vi "Translator.File.GetDefaultStrings (Single).vi"(5 "refnum in":T1, 7 "group":string, 8 "error in":errorcluster, 9 "label":string, 10 "default value":string) -> (0 "error out":errorcluster, 2 "value out":string)   [LabVIEW 2019, in "Tools.lvlib"]
uses:
  Tools.lvlib
  <vilib>/Utility/config.llb/Config Data RefNum.ctl
  <vilib>/Utility/config.llb/Read Key (String).vi
  <vilib>/Utility/config.llb/NI_LVConfig.lvlib
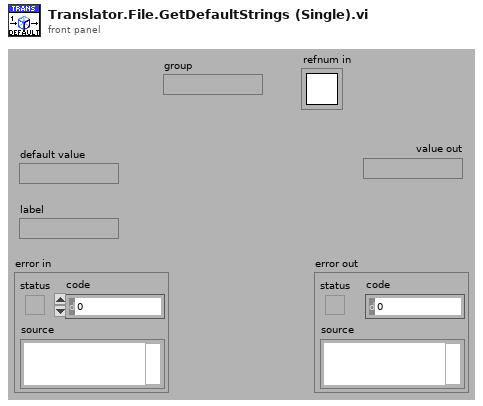
[diagram p1: front panel]
types:
  T1 = typedef "NI_LVConfig.lvlib/Config Data RefNum.ctl" = refnum<k1>
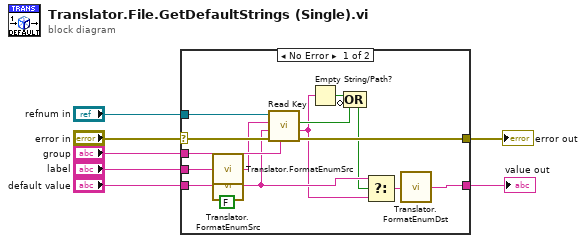
[diagram p0: block diagram]
diagram:
  n1 = case shown="No Error" "error in" {
    selector: "error in" -> [w18 w24]
    tunnel: "refnum in" -> [w17 _]
    tunnel: [w22 w24] -> w7
    tunnel: [w21 w23] -> w4
    tunnel: "group" -> [w20 _]
    tunnel: "label" -> [w16 _]
    tunnel: "default value" -> [w19 w23]
    frame No Error {
      n2 = call "Translator.FormatEnumSrc.vi"("text in"=w16) -> ("text out"=w9:string)  [unwired: 1 in]
      n3 = call "Translator.FormatEnumSrc.vi"("text in"=w19, "quotas?(T)"=FALSE) -> ("text out"=w15:string)
      n4 = call-poly <vilib>:"Read Key.vi"("section"=w20, "error in (no error)"=w18, "default value"=w15, "key"=w9, "refnum"=w17) -> ("error out"=w22:errorcluster, "value"=w11:string, "found?"=w12:bool)  [unwired: 3 in, 1 out]
      n5 = Empty String/Path?(string/path=w11) -> (empty?=w14:bool)
      n6 = Compound Arithmetic op=OR(w14, invert w12) -> (w13:bool)
      n7 = Select(t=w15, s=w13, f=w11) -> (s? t:f=w8:string)
      n8 = call "Translator.FormatEnumDst.vi"("text in"=w8) -> ("text out"=w21:string)
    }
    frame Error {
    }
  }
  "error out" <- w7
  "value out" <- w4
